vi "XNET Fill In Error Info.vi"(1 "depth (1)":i32=1, 5 "status code":i32, 7 "extended error info (empty)":string, 11 "error in":errorcluster) -> (15 "error out":errorcluster)   [LabVIEW 2018]
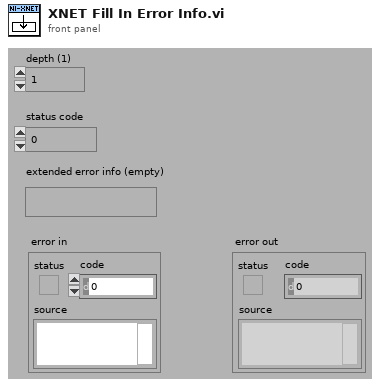
[diagram p1: front panel]
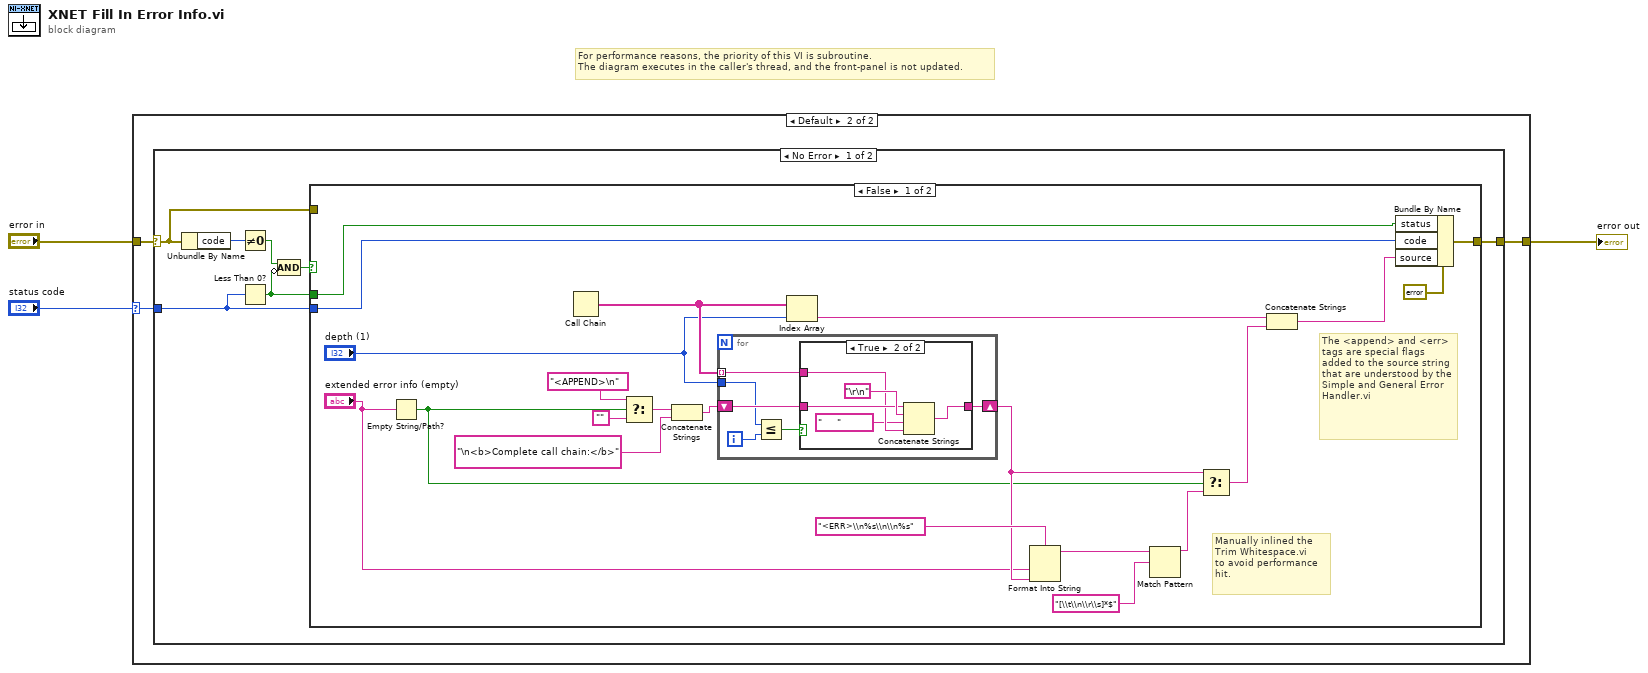
[diagram p0: block diagram]
diagram:
  # "For performance reasons, the priority of this VI is subroutine.\nThe diagram executes in the caller's thread, and the front-panel is not updated."
  n1 = case shown="Default" "status code" {
    selector: "status code" -> [_ w5]
    tunnel: [w4 w7] -> w3
    tunnel: "error in" -> [w4 w6]
    frame 0 {
      # "If the error code in equals zero, then propagate the error in cluster regardless of its value."
    }
    frame Default {
      n2 = case shown="No Error" w6 {
        selector: w6 -> [w12 w49]
        tunnel: [w14 w49] -> w7
        tunnel: w5 -> [w11 _]
        frame No Error {
          n3 = Unbundle By Name(w12) -> ("code"=w13:i32)
          n4 = Not Equal To 0?(x=w13) -> (x != 0?=w10:bool)
          n5 = Less Than 0?(x=w11) -> (x < 0?=w8:bool)
          n6 = Compound Arithmetic op=AND(w10, invert w8) -> (w9:bool)
          n7 = case shown="False" w9 {
            tunnel: [w35 w48] -> w14
            tunnel: w11 -> [w32 _]
            tunnel: w12 -> [_ w48]
            tunnel: w8 -> [w17 _]
            frame False {
              # "Manually inlined the\nTrim Whitespace.vi\nto avoid performance\nhit."
              # "The <append> and <err> tags are special flags added to the source string that are understood by the Simple and General Error Handler.vi"
              n8 = Empty String/Path?(string/path="extended error info (empty)") -> (empty?=w28:bool)
              n9 = Call Chain() -> (call chain=w16:string[])
              n10 = Select(t="<APPEND>\n", s=w28, f="") -> (s? t:f=w19:string)
              n11 = Concatenate Strings(w19, "\n<b>Complete call chain:</b>" ("call chain header")) -> (w22:string)
              n12 = for {
                tunnel: w16 -> [w39] mode=indexing
                shift-right: [w41] -> w30
                shift-left: w22 -> [w40]
                tunnel: "depth (1)" -> [w36]
                i -> [w37]
                n13 = Less Or Equal?(x=w36, y=w37) -> (x <= y?=w38:bool)
                n14 = case shown="True" w38 {
                  tunnel: [w42 w47] -> w41
                  tunnel: w40 -> [w42 w45]
                  tunnel: w39 -> [_ w44]
                  frame False {
                  }
                  frame True {
                    n15 = Concatenate Strings(w45, "\r\n", "     ", w44) -> (w47:string)
                  }
                }
              }
              n16 = Index Array(array=w16, index="depth (1)") -> (element=w24:string)
              n17 = Format Into String(format string="<ERR>\\n%s\\n\\n%s", "extended error info (empty)", w30) -> (resulting string=w26:string)  [unwired: 2 in, 1 out]
              n18 = Match Pattern(string=w26, regular expression="[\\t\\n\\r\\s]*$") -> (before substring=w25:string)  [unwired: 1 in, 3 out]
              n19 = Select(t=w30, s=w28, f=w25) -> (s? t:f=w29:string)
              n20 = Concatenate Strings(w24, w29) -> (w33:string)
              n21 = Bundle By Name(cluster=errorcluster {"status"=FALSE, "code"=0, "source"=""} ("error out"), "status"=w17, "code"=w32, "source"=w33) -> (w35:errorcluster)
            }
            frame True {
              # "If the error code input is setting a warning, and a warning is already set on the wire, then we\ngo with the one already on the wire."
            }
          }
        }
        frame Error {
          # "An error in trumps any error code input."
        }
      }
    }
  }
  "error out" <- w3
